vi "Setup SMU_PD and Measure Capacitance Only.vi"(0 "Semiconductor Module Context":T2, 1 "SMU_PD_Pin":string[](array[string])=["VDD"], 2 "Measurement Id":string="CMax", 3 "PD_v":dbl=41.0 format="%#_13g", 5 "error in (no error)":errorcluster, 6 "VNAs Measurement Parameters":T1) -> (14 "Semiconductor Module Context Out":T2, 19 "error out":errorcluster)   [LabVIEW 2013]
uses:
  <vilib>/NI_TestStand_SemiconductorModule/NI_TestStand_Semiconductor_Module.lvlibp/PinMap/General/SemiconductorModuleContext.ctl
  VNA/VNAs Measurement Parameters.ctl
  <vilib>/NI_TestStand_SemiconductorModule/NI_TestStand_Semiconductor_Module.lvlibp
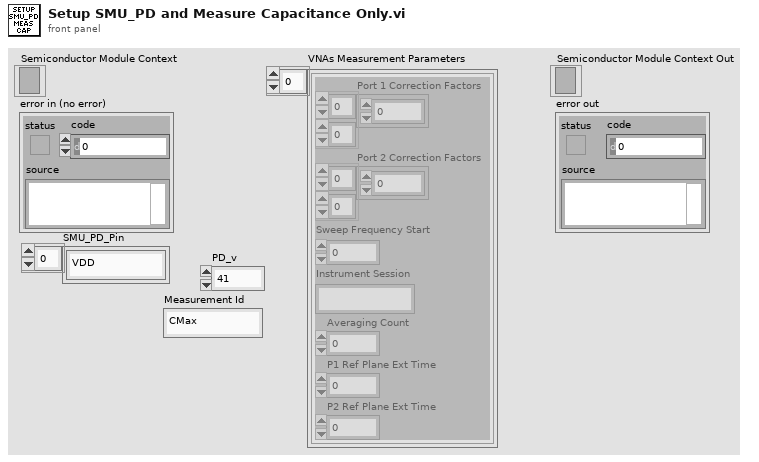
[diagram p1: front panel]
types:
  T1 = typedef "VNAs Measurement Parameters.ctl" = cluster{"Port 1 Correction Factors":cdb[][], "Port 2 Correction Factors":cdb[][], "Sweep Frequency Start":dbl, "Instrument Session":string, "Averaging Count":i32, "P1 Ref Plane Ext Time":dbl, "P2 Ref Plane Ext Time":dbl}[]
  T2 = typedef "NI_TestStand_Semiconductor_Module.lvlibp/SemiconductorModuleContext.ctl" = refnum<k7>
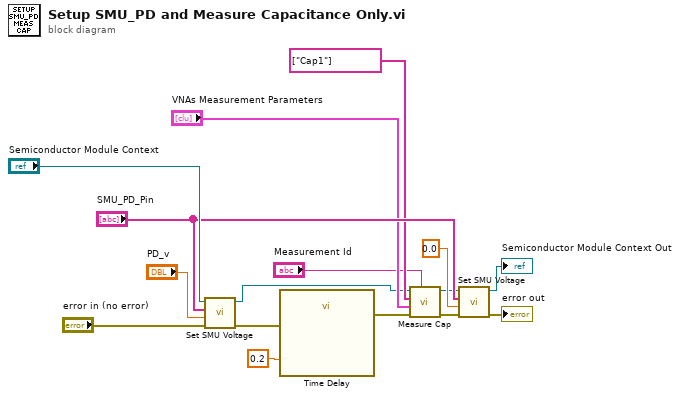
[diagram p0: block diagram]
diagram:
  n1 = call "Set SMU Voltage.vi"("error in (no error)"="error in (no error)", "VDD voltage level"="PD_v", "Pins"="SMU_PD_Pin", "Semiconductor Module Context"="Semiconductor Module Context") -> ("error out"=w11:errorcluster, "Semiconductor Module Context Out"=w2:T2)  [unwired: 5 in, 1 out]
  n2 = call "Time Delay"("error in (no error)"=w11, "Delay Time (s)"=0.2) -> ("error out"=w7:errorcluster)  [unwired: 9 in]
  n3 = call "Measure Cap.vi"("Measurement Id"="Measurement Id", "error in (no error)"=w7, "VNAs Measurement Parameters"="VNAs Measurement Parameters", "Pins"=string[] ["Cap1"] ("Capacitance Pins"), "Semiconductor Module Context"=w2) -> ("error out"=w6:errorcluster, "Semiconductor Module Context Out"=w1:T2)  [unwired: 4 in, 1 out]
  n4 = call "Set SMU Voltage.vi"("error in (no error)"=w6, "VDD voltage level"=0.0, "Pins"="SMU_PD_Pin", "Semiconductor Module Context"=w1) -> ("error out"=→"error out":errorcluster, "Semiconductor Module Context Out"=→"Semiconductor Module Context Out":T2)  [unwired: 5 in, 1 out]
